vi "Phase Uploaded.vi"(8 "error in (no error)":errorcluster, 11 "Cam_SLM_Controller in":refnum<class "Cam_SLM_Controller.lvclass">) -> (0 "error out":errorcluster, 3 "Cam_SLM_Controller out":refnum<class "Cam_SLM_Controller.lvclass">)   [LabVIEW 2023, in "Cam_SLM_controller.lvlib" / "Cam_SLM_Controller.lvclass"]
uses:
  Cam_SLM_Controller.lvclass
  Cam_SLM_Controller.lvclass/Cam_SLM_Controller.ctl
  <vilib>/ActorFramework/Message Enqueuer/Message Enqueuer.lvclass/Message Enqueuer.ctl
  <vilib>/ActorFramework/Message Enqueuer/Enqueue.vi
  UIs/Camera_Controller/Camera_Controller Messages/External_Acq Msg/External_Acq Msg.lvclass
  <vilib>/ActorFramework/Message Priority Queue/Priority Enqueue.vi
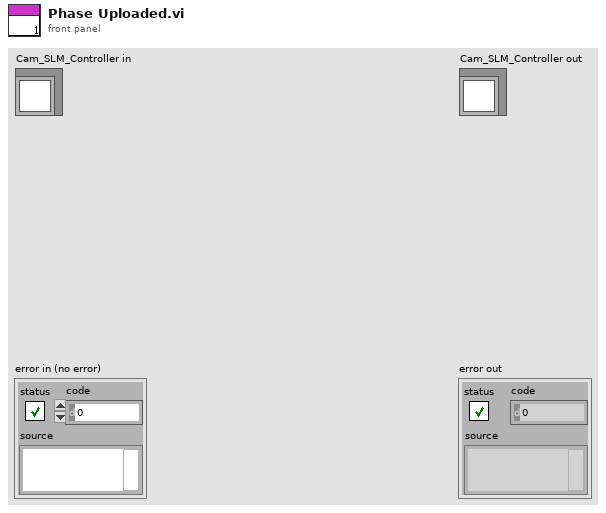
[diagram p1: front panel]
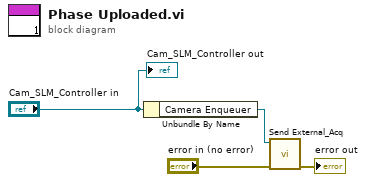
[diagram p0: block diagram]
diagram:
  n1 = Unbundle By Name("Cam_SLM_Controller in") -> ("Camera Enqueuer"=w3:refnum<class "Message Enqueuer.lvclass">)
  n2 = call "Send External_Acq.vi"("error in (no error)"="error in (no error)", "Message Enqueuer"=w3) -> ("error out"=→"error out":errorcluster)  [unwired: 8 in, 1 out]
  "Cam_SLM_Controller out" <- "Cam_SLM_Controller in"
